vi "Teach.vi"(0 "Neural Network In":refnum<class "Neural Network.lvclass">, 5 "Teaching File Path":path, 7 "Validation File Path":path, 9 "Settings":T1={"Max Epocs"=10000, "Max Time (s)"=10.0, "Error Goal (%)"=0.1, "# Vectors per Iteration"=200}, 11 "Error In":errorcluster) -> (4 "Neural Network Out":refnum<class "Neural Network.lvclass">, 6 "Teaching Time (s)":dbl, 8 "Solution Found":bool, 10 "% Error / Output":dbl[][](array[numeric]), 15 "Error Out":errorcluster)   [LabVIEW 2015, in "Neural Network.lvclass"]
doc: "Use RProp algorithm to teach the neural network based on the teaching and validation sets. Calculate scaling coeficients based on the input teaching vectors. The scaling coeficients will be used whenever you calculate the response of the network to some input.\n\n<b>Teaching File Path</b> - this is the set of teaching vectors that is the basis of teaching the network. Error evaluated over this network is back propagated through the network and is used to update the weights. \n\n<b>Validation File Path</b> - this set is not used to teach the network, only to stop the algorithm if the % error is smaller than the target for each output.\n\n<b>Settings</b> - maximum number of iterations of the algorithm, the target % error goal from 0 to 1, max time after which the algorithm will stop, and maximum memory chunk size read from teaching and validation files. The last value can be used to optimize behavior on systems with limited resources.\n\n<b>% Error / Output</b> -2D array output containing information about % error trend on each output. The % error value is calculated with the expected output being equal 100%.\n\n<b>Solution Found</b> - this indicator informs the user that a solution to the provided teaching samples has been found and the network is ready to operate correctly. This will be false if the teaching algorithm reaches maximum time or number of teaching iterations."
uses:
  Neural Network.lvclass
  Types/Teaching Settings.ctl
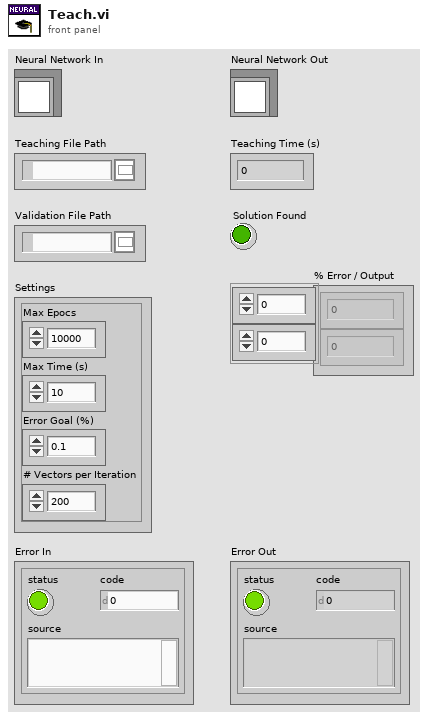
[diagram p1: front panel]
types:
  T1 = typedef "Neural Network.lvclass/Teaching Settings.ctl" = cluster{"Max Epocs":u64, "Max Time (s)":dbl, "Error Goal (%)":dbl, "# Vectors per Iteration":i64}
  T2 = typedef "Neural Network.lvclass/RProp Algorithm.ctl" = cluster{"Empty Gradient":T3[], "Gradient Register":T3[], "Teach Coef Register":T3[], "Current Gradient":T3[], "# Vectors per Iteration":i64, "Teaching Set Ref":refnum<k34>, "Validation Set Ref":refnum<k34>, "Error Buffer":dbl[], "# Samples":i64, "Gradient Sign Running Value":T3[]}
  T3 = typedef "Neural Network.lvclass/2D Array.ctl" = cluster{"2D Array":sgl[][]}
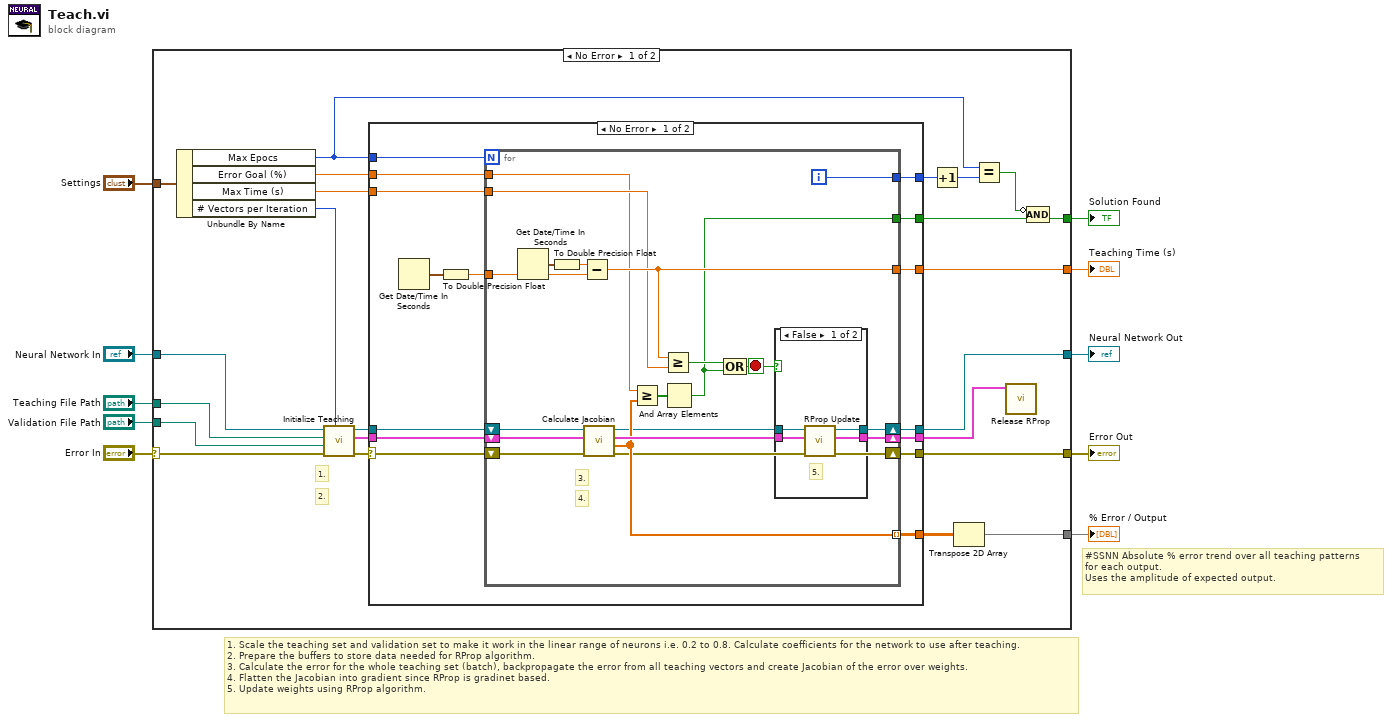
[diagram p0: block diagram]
diagram:
  # "#SSNN Absolute % error trend over all teaching patterns\nfor each output.\nUses the amplitude of expected output."
  # "1. Scale the teaching set and validation set to make it work in the linear range of neurons i.e. 0.2 to 0.8. Calculate coefficients for the network to use after teaching.\n2. Prepare the buffers to store data needed for RProp algorithm.\n3. Calculate the error for the whole teaching set (batch), backpropagate the error from all teaching vectors and create Jacobian of the error over weights.\n4. Flatten the Jacobian into gradient since RProp is gradinet based.\n5. Update weights using RProp algorithm."
  n1 = case shown="No Error" "Error In" {
    selector: "Error In" -> [w18 w78]
    tunnel: "Neural Network In" -> [w20 w79]
    tunnel: "Settings" -> [w33 _]
    tunnel: [w19 w79] -> w8
    tunnel: [w11 _] -> w1
    tunnel: [w25 _] -> w7
    tunnel: [w16 w78] -> w6
    tunnel: "Teaching File Path" -> [w24 _]
    tunnel: "Validation File Path" -> [w23 _]
    tunnel: [w13 _] -> w2
    frame No Error {
      # "2."
      # "1."
      n2 = Unbundle By Name(w33) -> ("Max Epocs"=w28:u64, "Error Goal (%)"=w32:dbl, "Max Time (s)"=w31:dbl, "# Vectors per Iteration"=w14:i64)
      n3 = call "Initialize Teaching.vi"("# Vectors per Iteration"=w14, "Error In"=w18, "Validation Set Path In"=w23, "Teaching Set Path In"=w24, "Neural Network In"=w20) -> ("Error Out"=w15:errorcluster, "RProp Data"=w22:T2, "Neural Network Out"=w21:refnum<class "Neural Network.lvclass">)  [unwired: 4 in]
      n4 = case shown="No Error" w15 {
        selector: w15 -> [w37 w75]
        tunnel: w32 -> [w48 _]
        tunnel: w31 -> [w47 _]
        tunnel: [w46 _] -> w12
        tunnel: [w45 _] -> w30
        tunnel: w28 -> [w44 _]
        tunnel: [w43 _] -> w26
        tunnel: w22 -> [w42 w76]
        tunnel: w21 -> [w41 w77]
        tunnel: [w40 w77] -> w19
        tunnel: [w39 w76] -> w17
        tunnel: [w38 w75] -> w16
        tunnel: [w34 _] -> w13
        frame No Error {
          n5 = Get Date/Time In Seconds() -> (seconds since 1Jan1904=w36:timestamp)
          n6 = To Double Precision Float(number=w36) -> (double precision float=w35:dbl)
          n7 = for {
            N: w44 -> [_]
            tunnel: w48 -> [w50]
            tunnel: [w55] -> w46 mode=indexing
            tunnel: w47 -> [w51]
            tunnel: [w49] -> w43
            tunnel: w35 -> [w65]
            tunnel: [w63] -> w45
            shift-right: [w56] -> w39
            shift-left: w42 -> [w60]
            shift-right: [w58] -> w40
            shift-left: w41 -> [w61]
            shift-right: [w54] -> w38
            shift-left: w37 -> [w59]
            tunnel: [w53] -> w34
            i -> [w63]
            stop <- w68 stop-if-true
            # "4."
            # "3."
            n8 = Get Date/Time In Seconds() -> (seconds since 1Jan1904=w67:timestamp)
            n9 = To Double Precision Float(number=w67) -> (double precision float=w66:dbl)
            n10 = Subtract(x=w66, y=w65) -> (x-y=w53:dbl)
            n11 = call "Calculate Jacobian.vi"("Error In"=w59, "RProp Data"=w60, "Neural Network In"=w61) -> ("Error Out"=w54:errorcluster, "Total % Error / Output"=w55:dbl[], "RProp Data Out"=w57:T2, "Neural Network Out"=w52:refnum<class "Neural Network.lvclass">)  [unwired: 5 in]
            n12 = Greater Or Equal?(x=w50, y=w55) -> (x >= y?=w62:bool[])
            n13 = Greater Or Equal?(x=w53, y=w51) -> (x >= y?=w64:bool)
            n14 = And Array Elements(Boolean array=w62) -> (logical AND=w49:bool)
            n15 = Compound Arithmetic op=OR(w64, w49) -> (w68:bool)
            n16 = case shown="False" w68 {
              tunnel: w52 -> [w71 w74]
              tunnel: [w72 w74] -> w58
              tunnel: w57 -> [w70 w73]
              tunnel: [w69 w73] -> w56
              frame False {
                # "5."
                n17 = call "RProp Update.vi"("RProp Data"=w70, "Neural Network In"=w71) -> ("RProp Data Out"=w69:T2, "Neural Network Out"=w72:refnum<class "Neural Network.lvclass">)  [unwired: 8 in]
              }
              frame True {
              }
            }
          }
        }
        frame Error {
        }
      }
      n18 = Increment(x=w30) -> (x+1=w29:i32)
      n19 = Transpose 2D Array(2D array=w12) -> (transposed array=w11:dbl[][])
      n20 = Equal?(x=w28, y=w29) -> (x = y?=w27:bool)
      n21 = call "Release RProp.vi"("RProp Data"=w17) -> ()  [unwired: 11 in]
      n22 = Compound Arithmetic op=AND(invert w27, w26) -> (w25:bool)
    }
    frame Error {
    }
  }
  "Neural Network Out" <- w8
  "Error Out" <- w6
  "% Error / Output" <- w1
  "Solution Found" <- w7
  "Teaching Time (s)" <- w2
